vi "FFT demo.vi"() -> ()   [LabVIEW 2009]
uses:
  <vilib>/measure/maspectr.llb/FFT Spectrum (Real-Im) for N Chan.vi
  <vilib>/measure/maspectr.llb/FFT Power Spectrum for N Chan.vi
  <vilib>/express/express analysis/Spectral/XNode/ExpressSpectralMeasurementsBlockNode.xnode
  <vilib>/express/express analysis/Spectral/Block/exnSpectralBlock spectral measurements RMS poly.vi
  <vilib>/express/express analysis/Spectral/Block/exnSpectralBlock spectral measurements RMS DDT.vi
  <vilib>/measure/NI_MAPro.lvlib
panel:
  in  "phi":dbl(slide) scale=-3.14..3.14
  out "imaginary part":T1(graph)
  in  "f":dbl(slide)=1.9591836734693877 scale=0.0..8.0
  in  "dt":dbl=0.125
  out "Power spectrum":cluster{"f0":dbl, "df":dbl, "magnitude":dbl[]}[](graph)
  out "Real parts":cluster{"f0":dbl, "df":dbl, "real part":dbl[]}[](graph)
  out "Waveform Graph":dynamicdata(graph)
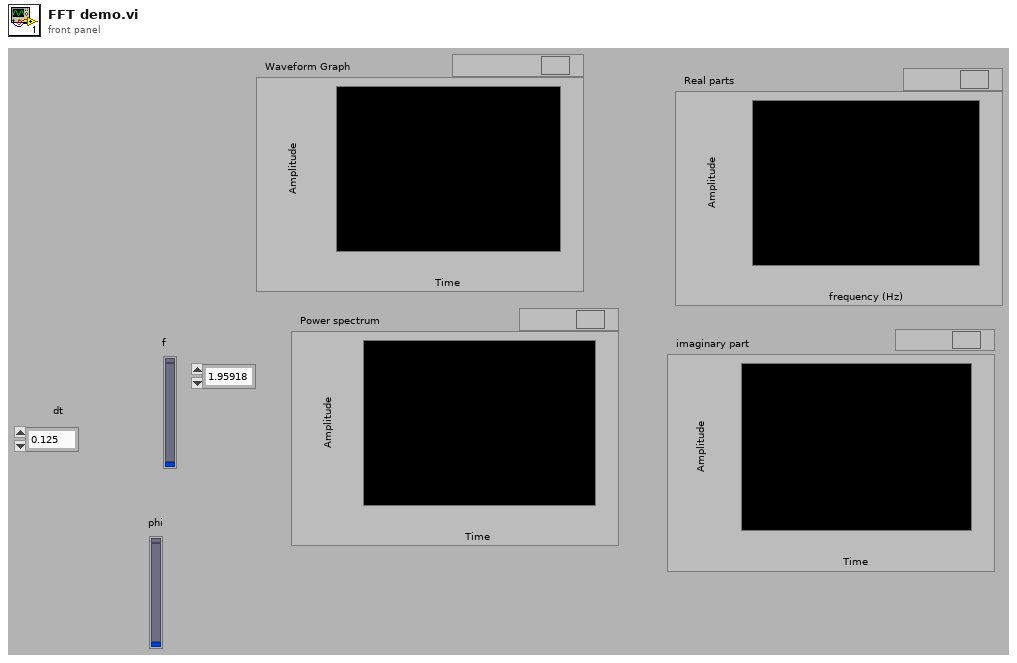
[diagram p1: front panel]
types:
  T1 = cluster{"f0":dbl, "df":dbl, "imaginary part":dbl[]}[]
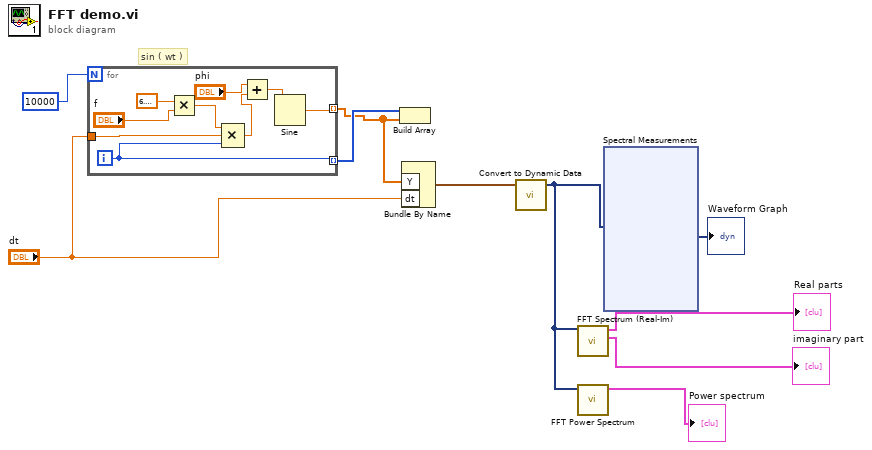
[diagram p0: block diagram]
diagram:
  # "sin ( wt )"
  n1 = for {
    N: 10000 -> [_]
    tunnel: [w19] -> w6 mode=indexing
    tunnel: [w18] -> w8 mode=indexing
    tunnel: "dt" -> [w17]
    i -> [w18]
    n2 = Multiply(x=6.283185307179586, y="f") -> (x*y=w14:dbl)
    n3 = Compound Arithmetic op=MULTIPLY(w14, w17, w18) -> (w12:dbl)
    n4 = Add(x="phi", y=w12) -> (x+y=w11:dbl)
    n5 = Sine(x=w11) -> (sin(x)=w19:dbl)
  }
  n6 = Build Array(w8, w6) -> ()  [unwired: 1 out]
  n7 = Bundle By Name("Y"=w6, "dt"="dt") -> (w7:waveform(dbl))  [unwired: 1 in]
  n8 = call "Convert to Dynamic Data"("Waveform"=w7) -> ("Dynamic Data Type"=w5:dynamicdata)  [unwired: 3 in]
  n9 = call-poly <vilib>:"FFT Spectrum (Real-Im).vi"("time signals"=w5) -> ("imaginary parts"=→"imaginary part":T1, "real parts"=→"Real parts":cluster{"f0":dbl, "df":dbl, "real part":dbl[]}[])  [unwired: 6 in, 3 out]
  n10 = call-poly <vilib>:"FFT Power Spectrum.vi"("time signals"=w5) -> ("power spectra"=→"Power spectrum":cluster{"f0":dbl, "df":dbl, "magnitude":dbl[]}[])  [unwired: 7 in, 3 out]
  n11 = xnode "Spectral Measurements"("Signals"=w5) -> ("FFT - (RMS)"=→"Waveform Graph":dynamicdata)  [unwired: 1 in, 2 out]
